vi "GetSettings.vi"(8 "error in (no error)":errorcluster, 11 "configuration file path":path) -> (0 "error out":errorcluster, 3 "Settings":T1)   [LabVIEW 2013]
uses:
  TypeDef/Settings.ctl
  <vilib>/Utility/config.llb/Read Key (String).vi
  <vilib>/Utility/config.llb/NI_LVConfig.lvlib
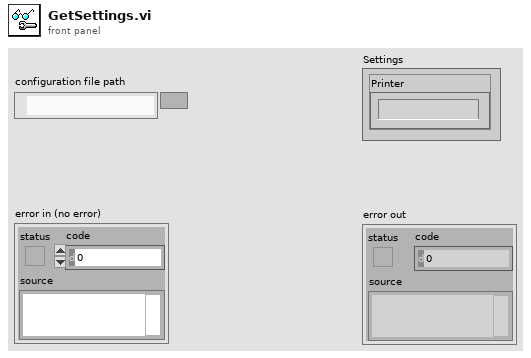
[diagram p1: front panel]
types:
  T1 = typedef "Settings.ctl" = cluster{"Printer":string}
  T2 = typedef "NI_LVConfig.lvlib/Config Data RefNum.ctl" = refnum<k1>
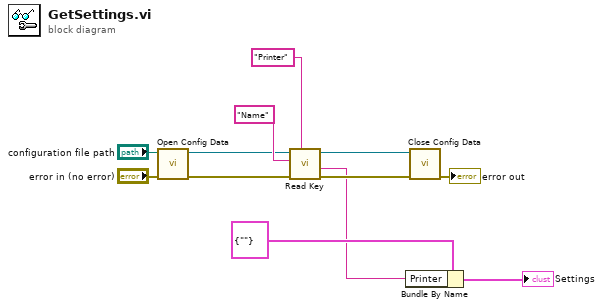
[diagram p0: block diagram]
diagram:
  n1 = call <vilib>:"Open Config Data.vi"("error in (no error)"="error in (no error)", "configuration file path"="configuration file path") -> ("error out"=w10:errorcluster, "refnum"=w9:T2)  [unwired: 7 in, 1 out]
  n2 = call-poly <vilib>:"Read Key.vi"("section"="Printer", "error in (no error)"=w10, "key"="Name", "refnum"=w9) -> ("error out"=w7:errorcluster, "value"=w4:string, "refnum out"=w8:T2)  [unwired: 4 in, 1 out]
  n3 = Bundle By Name(cluster=T1 {"Printer"=""}, "Printer"=w4) -> (→"Settings":T1)
  n4 = call <vilib>:"Close Config Data.vi"("error in (no error)"=w7, "refnum"=w8) -> ("error out"=→"error out":errorcluster)  [unwired: 8 in, 1 out]
